vi "Untitled 10 (SubVI).vi"(10 "см. 1.5 in":dbl[](array[numeric]), 11 "Кол-во выборок":i32=400) -> (3 "Pulse Pattern":dbl[](array[numeric]))   [LabVIEW 2017]
uses:
  <vilib>/Analysis/NI_AALBase.lvlib
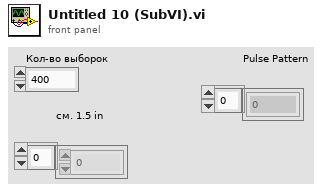
[diagram p1: front panel]
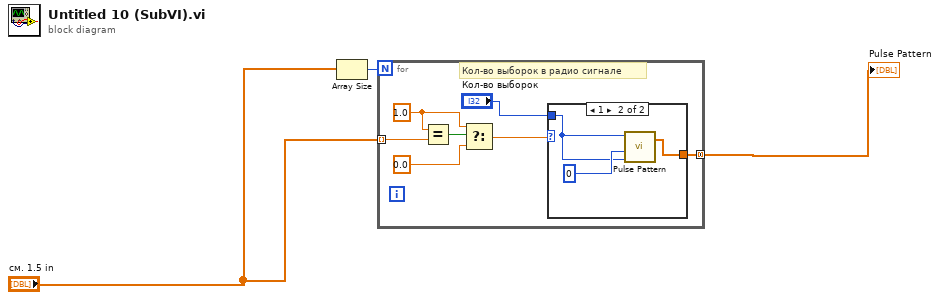
[diagram p0: block diagram]
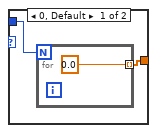
[diagram p2: hidden frame]
diagram:
  n1 = Array Size(array="см. 1.5 in") -> (size(s)=w1:i32)
  n2 = for {
    N: w1 -> [_]
    tunnel: [w6] -> w2 mode=concatenating
    tunnel: "см. 1.5 in" -> [w4] mode=indexing
    w9 = 1.0
    # "Кол-во выборок в радио сигнале"
    n3 = Equal?(x=w9, y=w4) -> (x = y?=w10:bool)
    n4 = Select(t=w9, s=w10, f=0.0) -> (s? t:f=w7:dbl)
    n5 = case shown="1" w7 {
      tunnel: [w11 w15] -> w6
      tunnel: "Кол-во выборок" -> [w12 w14]
      frame 0, Default {
        n6 = for {
          N: w12 -> [_]
          tunnel: [0.0] -> w11 mode=indexing
        }
      }
      frame 1 {
        n7 = call <vilib>:"Pulse Pattern.vi"("width"=w14, "delay"=0, "samples"=w14) -> ("Pulse Pattern"=w15:dbl[])  [unwired: 1 in, 1 out]
      }
    }
  }
  "Pulse Pattern" <- w2
